vi "Create.vi"(8 "error in":errorcluster, 10 "reset":bool, 11 "serial configuration":T1) -> (0 "error out":errorcluster, 3 "instrument out":refnum<class "Instrument.lvclass">)   [LabVIEW 2020, in "MeasurementLink 34401.lvlib" / "Instrument.lvclass"]
uses:
  Instrument.lvclass
  Instrument.lvclass/Instrument.ctl
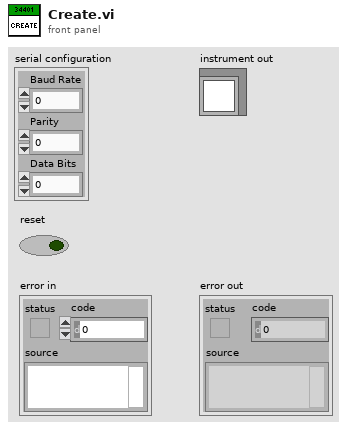
[diagram p1: front panel]
types:
  T1 = cluster{"Baud Rate":u32, "Parity":u16, "Data Bits":u16}
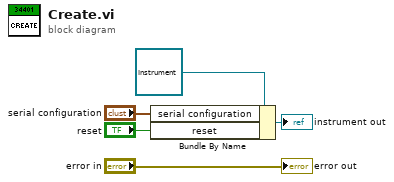
[diagram p0: block diagram]
diagram:
  n1 = Bundle By Name(cluster=refnum<class "Instrument.lvclass"> refnum ("Instrument in"), "serial configuration"="serial configuration", "reset"="reset") -> (→"instrument out":refnum<class "Instrument.lvclass">)
  "error out" <- "error in"
